vi "GT_SetDoBit.vi"(8 "Value":bool, 9 "doIndex":i16, 10 "doType":i16(ring) items=["MC_Enable", "MC_Clear", "MC_Gpo"], 11 "rtn_In":cluster{"rtn":i16, "Func":string}) -> (3 "rtn_Out":cluster{"rtn":i16, "Func":string})   [LabVIEW 2014]
uses:
  VC6/gts.dll
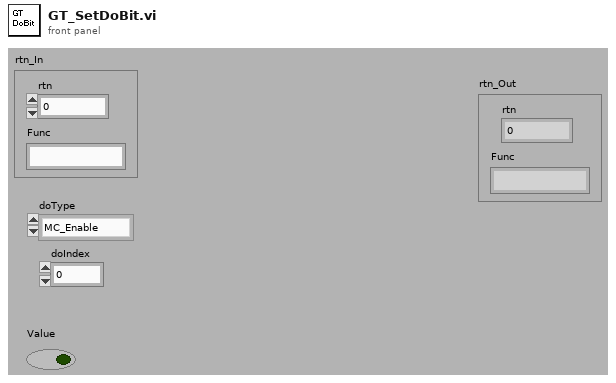
[diagram p1: front panel]
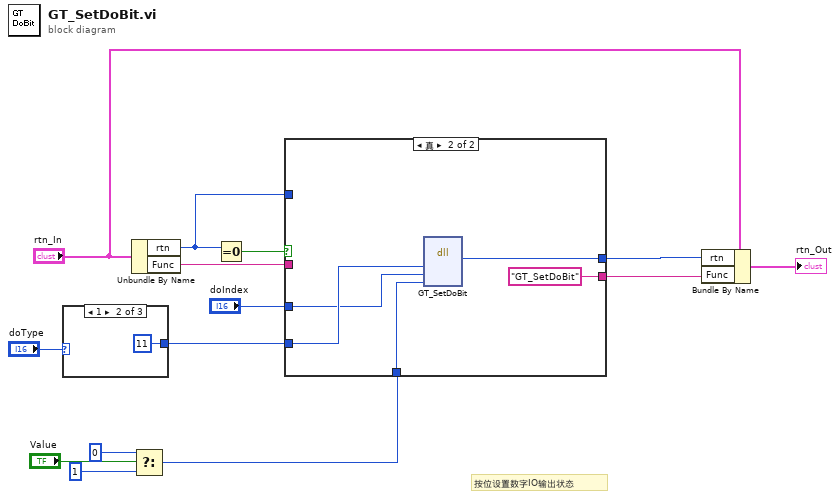
[diagram p0: block diagram]
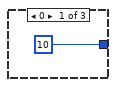
[diagram p2: hidden frame]
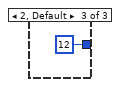
[diagram p3: hidden frame]
diagram:
  # "按位设置数字IO输出状态"
  n1 = case shown="1" "doType" {
    tunnel: [i16 10 ("doType") i16 11 ("doType") i16 12 ("doType")] -> w8
    frame 0 {
    }
    frame 1 {
    }
    frame 2, Default {
    }
  }
  n2 = Unbundle By Name("rtn_In") -> ("rtn"=w6:i16, "Func"=w7:string)
  n3 = Select(t=i16 0, s="Value", f=i16 1) -> (s? t:f=w1:i16)
  n4 = Equal To 0?(x=w6) -> (x = 0?=w14:bool)
  n5 = case shown="真" w14 {
    tunnel: [w18 w24] -> w11
    tunnel: [w19 "GT_SetDoBit" ("Func")] -> w10
    tunnel: w8 -> [_ w22]
    tunnel: w7 -> [w19 _]
    tunnel: w6 -> [w18 _]
    tunnel: "doIndex" -> [_ w21]
    tunnel: w1 -> [_ w20]
    frame False {
    }
    frame True {
      n6 = dll-call lib="PTH2Fabs DNewGTS AC-800LWin7版源程序-20170926gts85VC6gts.dll" fn="GT_SetDoBit"("doType"=w22, "doIndex"=w21, "value"=w20) -> ("rtn"=w24:i16)  [unwired: 6 in, 2 out]
    }
  }
  n7 = Bundle By Name(cluster="rtn_In", "rtn"=w11, "Func"=w10) -> (→"rtn_Out":cluster{"rtn":i16, "Func":string})
